vi "APX Monitor EPICS.vi"() -> ()   [LabVIEW 2015]
uses:
  <vilib>/Platform/TimedLoop/XDataNode/timing_clust.ctl
  <vilib>/Platform/TimedLoop/XDataNode/nitl_modes.ctl
  <vilib>/Platform/TimedLoop/XDataNode/wakeup.ctl
  <userlib>/caLab/Private/Get_PV-1D.vi
  <userlib>/caLab/Private/Put_I16-1D_PV-1D.vi
  <vilib>/platform/TimedLoop/XDataNode/XDataNode.xnode
  <vilib>/Platform/TimedLoop/XDataNode/XDNodeRunTimeDep.lvlib
panel:
  out "L2Turbo_ST":bool
  out "AP2Turbo_ST":bool
  out "HEMTurbo_ST":bool
  out "String":string
  out "APX:PREP_ILK":bool
  in  "OFFLINE/ONLINE":bool
  in  "APX_V1_CLOSE":bool
  in  "APX_V1_OPEN":bool
  in  "APX_V2_CLOSE":bool
  in  "APX_V2_OPEN":bool
  in  "APX_V3_CLOSE":bool
  in  "APX_V3_OPEN":bool
  in  "APX_V5_CLOSE":bool
  in  "APX_V5_OPEN":bool
  in  "APX_V4_CLOSE":bool
  in  "APX_V4_OPEN":bool
  in  "APX:Omniax:.VELO":dbl
  in  "APX:Omniax.ACCL":dbl
  in  "APX:OmniaxZ.SPMG":bool
  in  "APX:OmniaxZ.VAL":dbl
  in  "APX:Omniax:.TWV":dbl
  in  "APX:OmniaxX.TWR":bool
  in  "APX:OmniaxX.TWF":bool
  in  "APX:OmniaxY:.VELO":dbl
  in  "APX:OmniaxY.ACCL":dbl
  in  "APX:OmniaxY.SPMG":bool
  in  "APX:OmniaxY.VAL":dbl
  in  "APX:Omniaxy:.TWV":dbl
  in  "APX:OmniaxY.TWR":bool
  in  "APX:OmniaxY.TWF":bool
  in  "APX:OmniaxX:.VELO":dbl
  in  "APX:OmniaxX.ACCL":dbl
  in  "APX:OmniaxX.SPMG":bool
  in  "APX:OmniaxX.VAL":dbl
  in  "APX:Omniaxx:.TWV":dbl
  in  "APX:OmniaxX.TWR":bool
  in  "APX:OmniaxX.TWF":bool
  out "BL13-2:IG1Pressure":dbl format="%.2e"
  out "APX:HEMTurboF":dbl
  out "APX:HEMTurboP":dbl
  out "APX:HEMturboS":string
  out "APX:L2TurboF":dbl
  out "APX:L2TurboP":dbl
  out "APX:L2TurboS":string
  out "APX:AP2TurboF":dbl
  out "APX:AP2TurboP":dbl
  out "APX:AP2TurboS":string
  out "APX:V3_ENB":bool
  out "APX:V3_OPEN_REQ":bool
  out "APX:V3_SCL":bool
  out "APX:V3_SOP":bool
  out "BL132_ILK":bool
  out "SES-100_ILK":bool
  in  "loop":u8
  out "APX:V2_ENB":bool
  out "APX:V5_ENB":bool
  out "APX:V1_ENB":bool
  out "APX:V7_ENB":bool
  out "APX:V0_ENB":bool
  out "APX:V6_ENB":bool
  out "APX:V4_ENB":bool
  out "APX:V5_OPEN_REQ":bool
  out "APX:V2_OPEN_REQ":bool
  out "APX:V1_OPEN_REQ":bool
  in  "APX:V6_OPEN_REQ":bool
  out "APX:V4_OPEN_REQ":bool
  in  "APX:V0_OPEN_REQ":bool
  in  "APX:V7_OPEN_REQ":bool
  out "APX:V7_SCL":bool
  out "APX:V7_SOP":bool
  out "APX:V0_SCL":bool
  out "APX:V0_SOP":bool
  out "APX:V5_SCL":bool
  out "APX:V5_SOP":bool
  out "APX:V1_SCL":bool
  out "APX:V1_SOP":bool
  out "APX:V6_SCL":bool
  out "APX:V6_SOP":bool
  out "APX:V4_SCL":bool
  out "APX:V4_SOP":bool
  out "APX:V2_SCL":bool
  out "APX:V2_SOP":bool
  out "APX:PiezoZ":dbl format="%#_3g"
  out "APX:PiezoY":dbl format="%#_3g"
  out "APX:PiezoX":dbl format="%#_3g"
  out "APX:OmniaxX":dbl format="%#_5g"
  out "APX:OmniaxY":dbl format="%#_5g"
  out "APX:OmniaxZ.RBV":dbl
  out "BL132:132WRG1":dbl format="%.2e"
  out "APX:HPC":dbl format="%.2e"
  out "APX:Tsample":dbl format="%.1f"
  out "APX:Tpiezo":dbl format="%.1f"
  out "APX:Thpc":dbl format="%.1f"
  out "APX LEN2":dbl format="%.2e"
  out "APX:AP2":dbl format="%.2e"
  out "APX:AP1":dbl format="%.2e"
  out "APX:PREP":dbl format="%.2e"
  out "APX:HPC100":dbl format="%.4f"
  in  "stop":bool
  out "APX:HPC01":dbl format="%.6g"
  # "APX EPICS"
  # "HEMTurbo"
  # "4"
  # "SES-100 Analyzer"
  # "300l/s"
  # "L2Turbo"
  # "70l/s"
  # "3"
  # "300l/s"
  # "AP2Turbo"
  # "2"
  # "500l/s"
  # "5"
  # "300l/s"
  # "BPTrubo"
  # "AP1Turbo"
  # "1"
  # "70l/s"
  # "300l/s"
  # "70l/s"
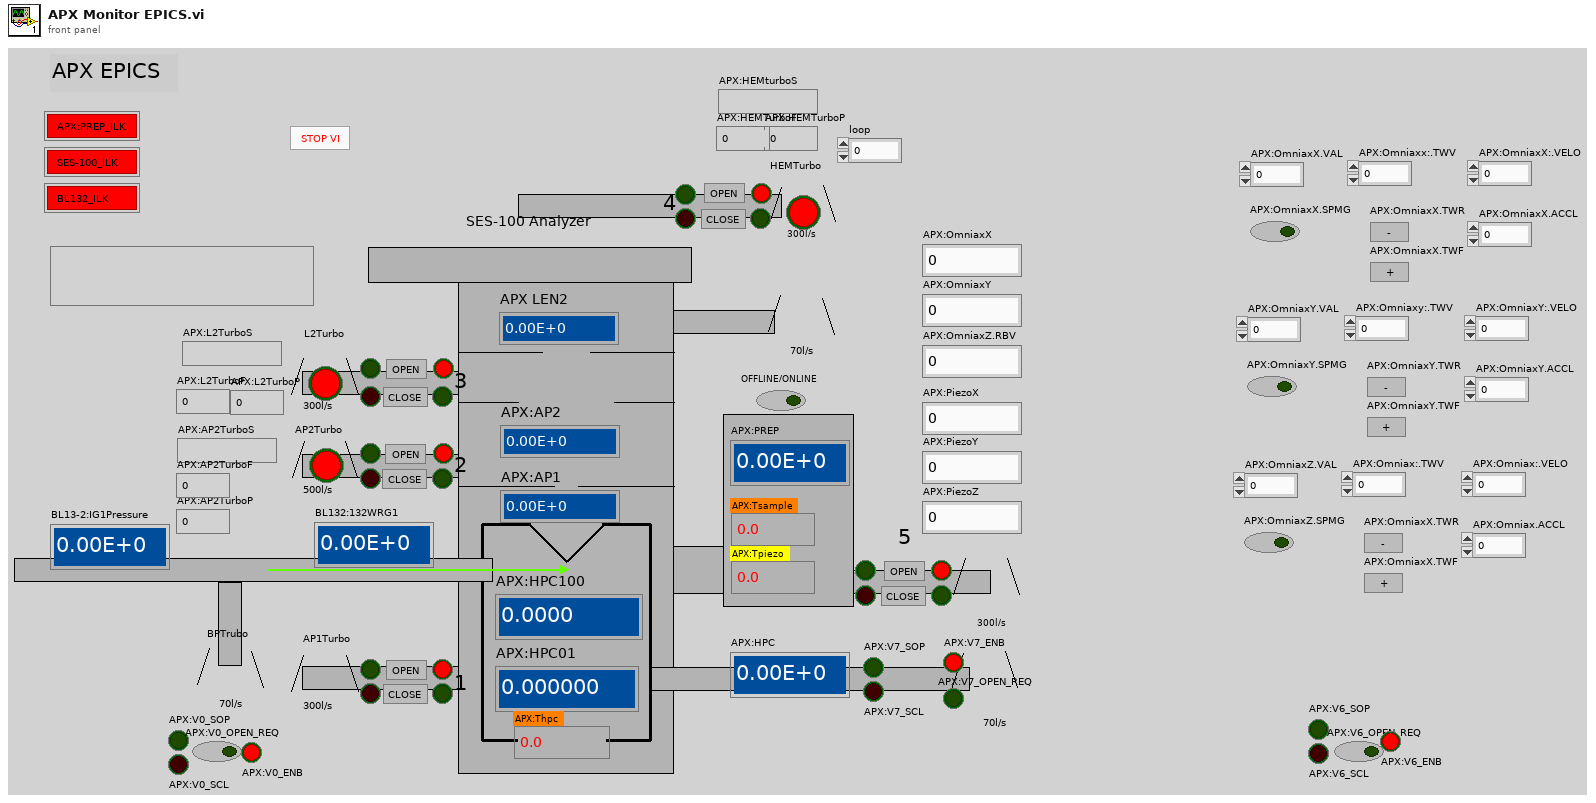
[diagram p1: front panel]
types:
  T1 = typedef "XDNodeRunTimeDep.lvlib/timing_clust.ctl" = cluster{"Expected End [f-1]":u64, "Actual End [f-1]":u64, "Finished Late? [f-1]":bool, "Expected End [i-1]":u64, "Actual End [i-1]":u64, "Finished Late? [i-1]":bool, "Expected Start [i]":u64, "Actual Start [i]":u64, "Expected Start [f]":u64, "Actual Start [f]":u64, "Source Name":string, "Structure Name":string, "Period":i64, "Deadline":i64, "Offset":i64, "Start":i64, "Priority":i32, "Timeout":i32, "Mode":T2, "Wakeup Reason":T3, "Error":errorcluster, "Source Type":string, "Secondary Source Type":string, "Global End Time":u64, "Global Start Time":u64, "Frame Duration":u64, "Iteration Duration":u64, "Assigned CPU":i32, "I/O Scan Engine Mode":u32}
  T2 = typedef "XDNodeRunTimeDep.lvlib/nitl_modes.ctl" = enum32{"No Change", "Process missed periods, maintain original phase", "Discard missed periods, maintain original phase", "Process missed periods, ignore original phase", "Discard missed periods, ignore original phase"}
  T3 = typedef "XDNodeRunTimeDep.lvlib/wakeup.ctl" = enum32{"Normal", "Aborted", "Asynchronous wakeup", "Timing source error", "Timed loop error", "Timeout"}
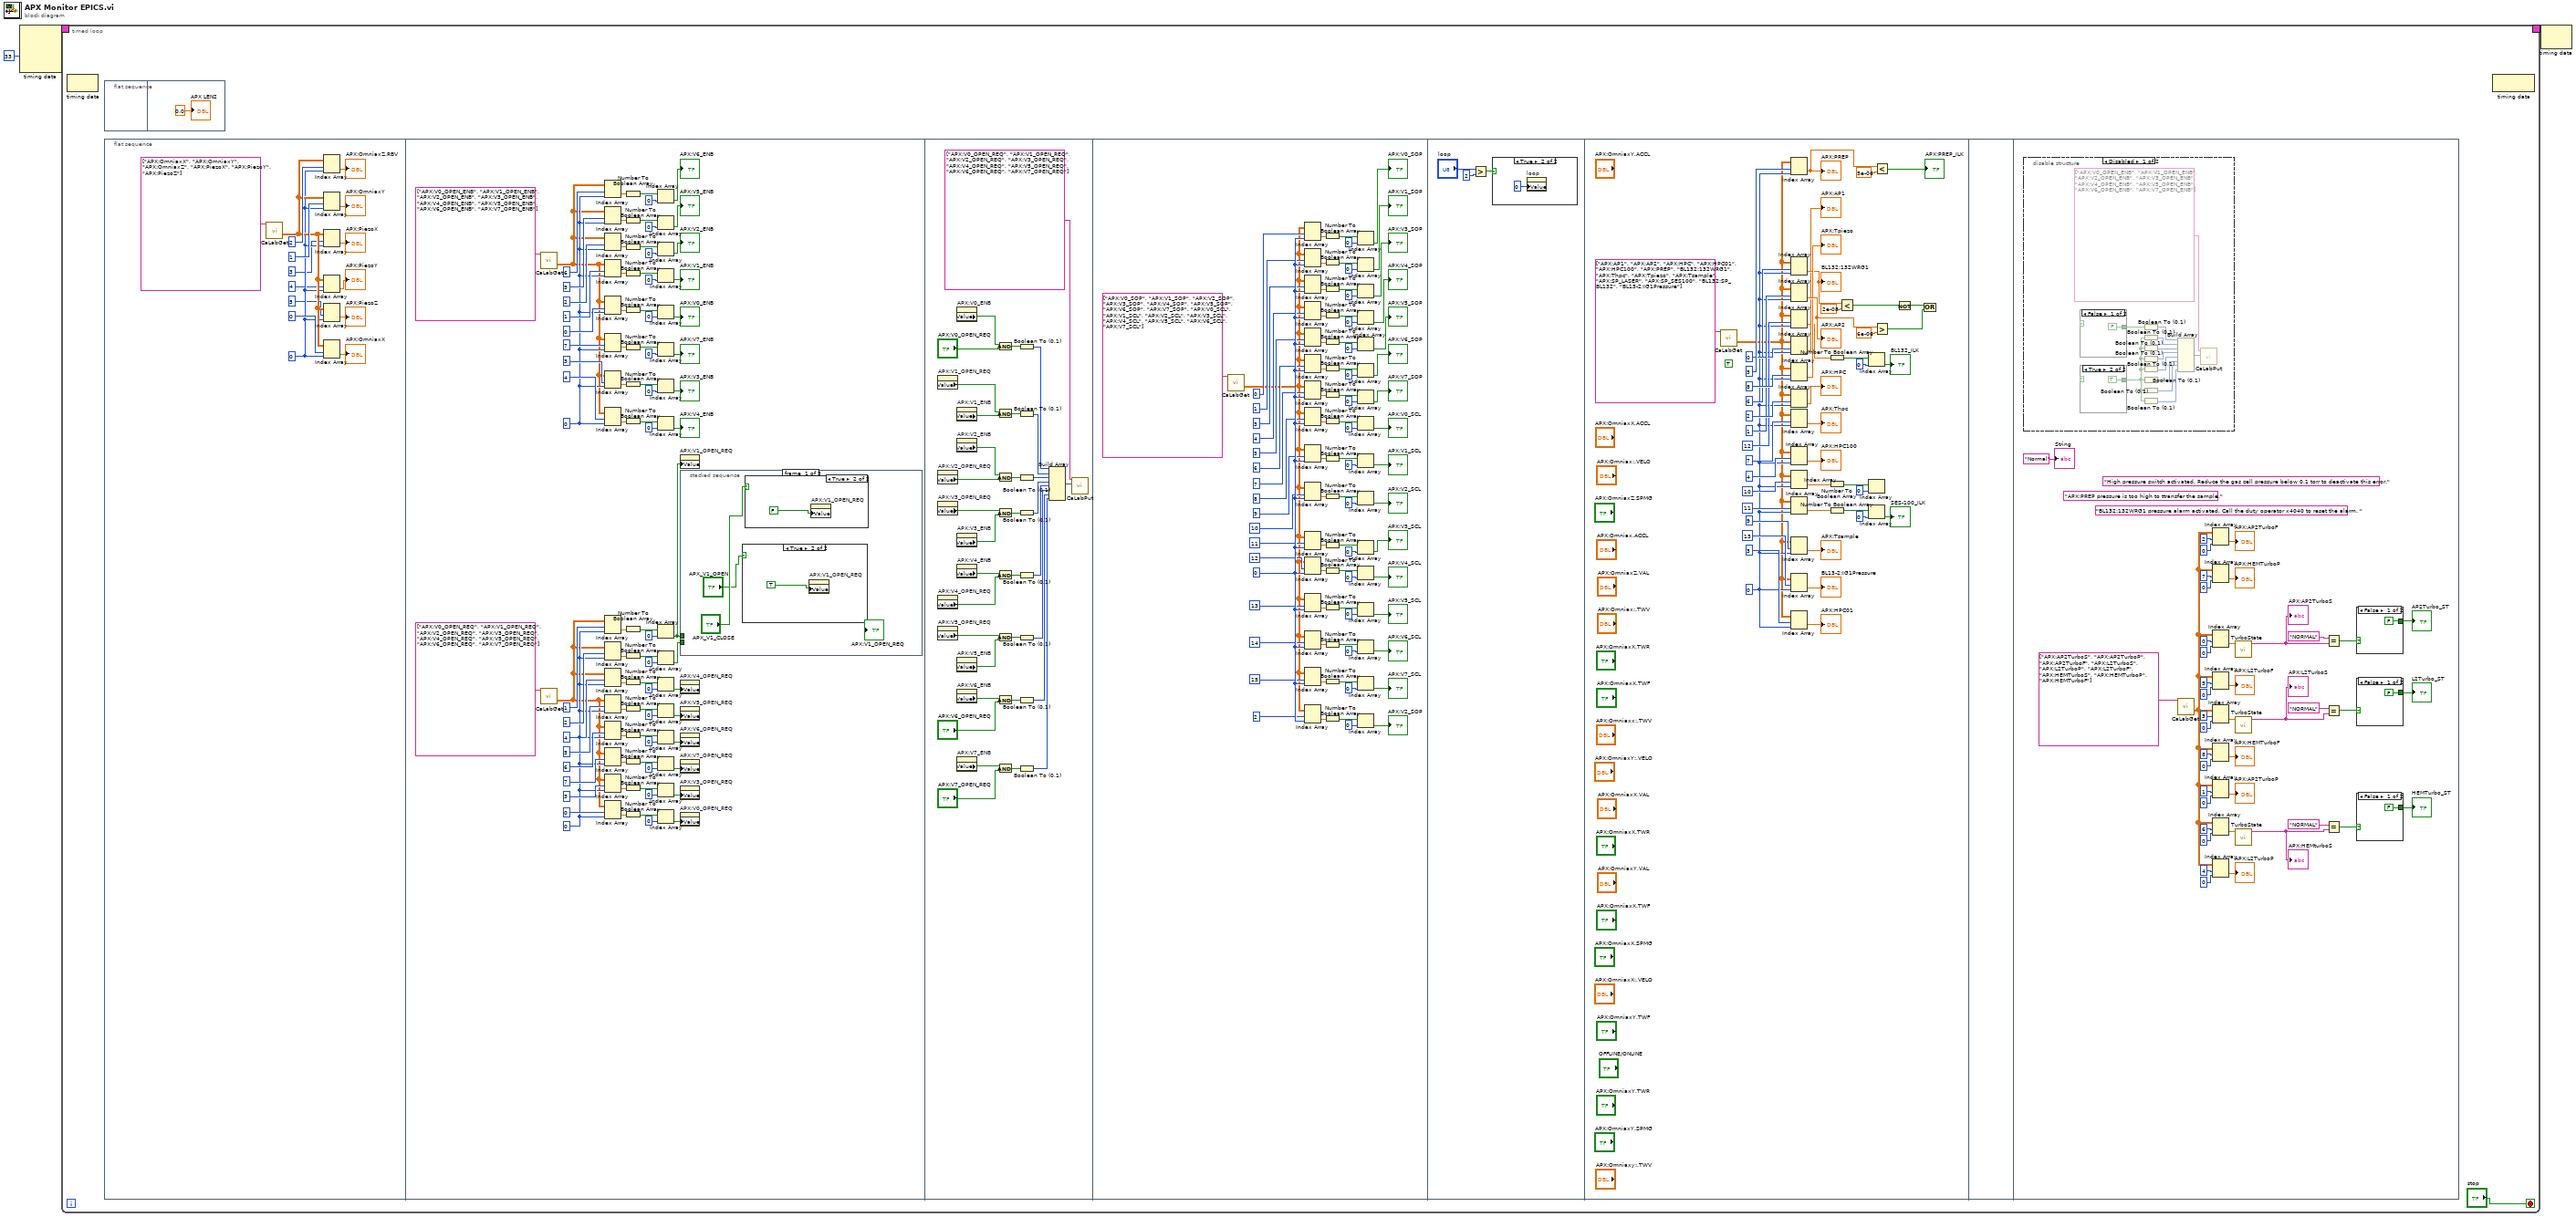
[diagram p0: block diagram]
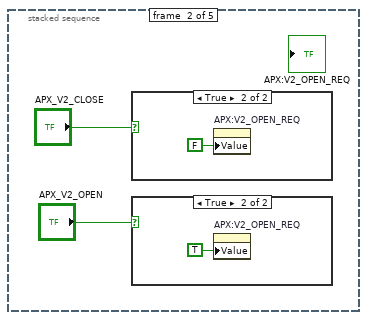
[diagram p4: hidden frame]
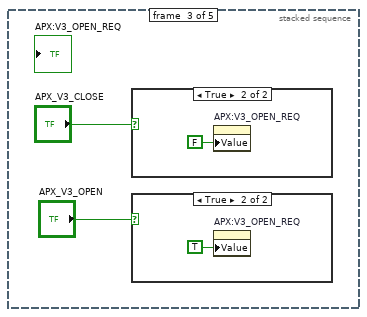
[diagram p7: hidden frame]
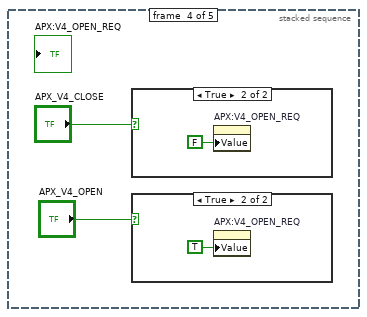
[diagram p10: hidden frame]
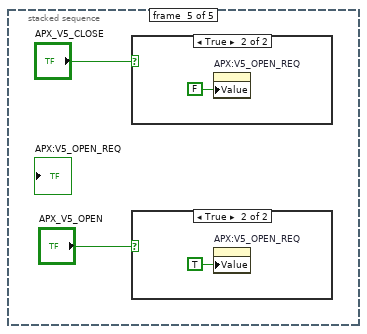
[diagram p13: hidden frame]
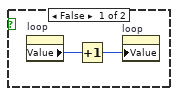
[diagram p16: hidden frame]
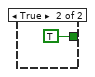
[diagram p17: hidden frame]
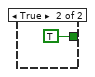
[diagram p18: hidden frame]
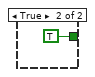
[diagram p19: hidden frame]
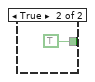
[diagram p20: hidden frame]
diagram:
  n1 = node-c288(33 ("Priority")) -> (w3:T1)  [unwired: 3 in]
  n2 = timed-loop {
    timing: w3 -> [_]
    timing-out: [_] -> w2
    stop <- "stop" stop-if-true
    n3 = node-c288() -> ()  [unwired: 1 in, 1 out]
    n4 = flat-sequence {
      frame #0 {
      }
      frame #1 {
        "APX LEN2" <- 0.0 ("APX LEN2")
      }
    }
    n5 = flat-sequence {
      frame #0 {
        w11 = 0 ("index")
        n6 = call-poly "CaLabGet.vi"("PV Names"=string[] ["APX:OmniaxX", "APX:OmniaxY", "APX:OmniaxZ", "APX:PiezoX", "APX:PiezoY", "APX:PiezoZ"]) -> ("Value Array (number)"=w12:dbl[][])  [unwired: 8 in, 6 out]
        n7 = Index Array(array=w12, index (row)=2, index (col)=w11) -> (element=→"APX:OmniaxZ.RBV":dbl)
        n8 = Index Array(array=w12, index (row)=1, index (col)=w11) -> (element=→"APX:OmniaxY":dbl)
        n9 = Index Array(array=w12, index (row)=3 ("disabled index (row)"), index (col)=w11) -> (element=→"APX:PiezoX":dbl)
        n10 = Index Array(array=w12, index (row)=4 ("disabled index (row)"), index (col)=w11) -> (element=→"APX:PiezoY":dbl)
        n11 = Index Array(array=w12, index (row)=5 ("disabled index (row)"), index (col)=w11) -> (element=→"APX:PiezoZ":dbl)
        n12 = Index Array(array=w12, index (row)=0, index (col)=w11) -> (element=→"APX:OmniaxX":dbl)
      }
      frame #1 {
        w53 = 0 ("index")
        w97 = 0 ("index")
        n13 = call-poly "CaLabGet.vi"("PV Names"=string[] ["APX:V0_OPEN_ENB", "APX:V1_OPEN_ENB", "APX:V2_OPEN_ENB", "APX:V3_OPEN_ENB", "APX:V4_OPEN_ENB", "APX:V5_OPEN_ENB", "APX:V6_OPEN_ENB", "APX:V7_OPEN_ENB"]) -> ("Value Array (number)"=w96:dbl[][])  [unwired: 8 in, 6 out]
        n14 = call-poly "CaLabGet.vi"("PV Names"=string[] ["APX:V0_OPEN_REQ", "APX:V1_OPEN_REQ", "APX:V2_OPEN_REQ", "APX:V3_OPEN_REQ", "APX:V4_OPEN_REQ", "APX:V5_OPEN_REQ", "APX:V6_OPEN_REQ", "APX:V7_OPEN_REQ"]) -> ("Value Array (number)"=w52:dbl[][])  [unwired: 8 in, 6 out]
        n15 = Index Array(array=w96, index (row)=6, index (col)=w97) -> (element=w73:dbl)
        n16 = Index Array(array=w96, index (row)=5, index (col)=w97) -> (element=w74:dbl)
        n17 = Index Array(array=w96, index (row)=2, index (col)=w97) -> (element=w77:dbl)
        n18 = Index Array(array=w96, index (row)=1, index (col)=w97) -> (element=w78:dbl)
        n19 = Index Array(array=w96, index (row)=0 ("disabled index (row)"), index (col)=w97) -> (element=w79:dbl)
        n20 = Index Array(array=w96, index (row)=7, index (col)=w97) -> (element=w72:dbl)
        n21 = Index Array(array=w96, index (row)=3, index (col)=w97) -> (element=w76:dbl)
        n22 = Index Array(array=w96, index (row)=4, index (col)=w97) -> (element=w75:dbl)
        n23 = Index Array(array=w52, index (row)=1, index (col)=w53) -> (element=w34:dbl)
        n24 = Index Array(array=w52, index (row)=2, index (col)=w53) -> (element=w33:dbl)
        n25 = Index Array(array=w52, index (row)=4, index (col)=w53) -> (element=w31:dbl)
        n26 = Index Array(array=w52, index (row)=5, index (col)=w53) -> (element=w30:dbl)
        n27 = Index Array(array=w52, index (row)=6, index (col)=w53) -> (element=w29:dbl)
        n28 = Index Array(array=w52, index (row)=7, index (col)=w53) -> (element=w28:dbl)
        n29 = Index Array(array=w52, index (row)=3, index (col)=w53) -> (element=w32:dbl)
        n30 = Index Array(array=w52, index (row)=0 ("disabled index (row)"), index (col)=w53) -> (element=w35:dbl)
        n31 = Number To Boolean Array(number=w73) -> (Boolean array=w83:bool[])
        n32 = Number To Boolean Array(number=w74) -> (Boolean array=w85:bool[])
        n33 = Number To Boolean Array(number=w77) -> (Boolean array=w91:bool[])
        n34 = Number To Boolean Array(number=w78) -> (Boolean array=w93:bool[])
        n35 = Number To Boolean Array(number=w79) -> (Boolean array=w95:bool[])
        n36 = Number To Boolean Array(number=w72) -> (Boolean array=w81:bool[])
        n37 = Number To Boolean Array(number=w76) -> (Boolean array=w89:bool[])
        n38 = Number To Boolean Array(number=w75) -> (Boolean array=w87:bool[])
        n39 = Number To Boolean Array(number=w34) -> (Boolean array=w49:bool[])
        n40 = Number To Boolean Array(number=w33) -> (Boolean array=w47:bool[])
        n41 = Number To Boolean Array(number=w31) -> (Boolean array=w43:bool[])
        n42 = Number To Boolean Array(number=w30) -> (Boolean array=w41:bool[])
        n43 = Number To Boolean Array(number=w29) -> (Boolean array=w39:bool[])
        n44 = Number To Boolean Array(number=w28) -> (Boolean array=w37:bool[])
        n45 = Number To Boolean Array(number=w32) -> (Boolean array=w45:bool[])
        n46 = Number To Boolean Array(number=w35) -> (Boolean array=w51:bool[])
        n47 = Index Array(array=w83, index=0) -> (element=→"APX:V6_ENB":bool)
        n48 = Index Array(array=w85, index=0) -> (element=→"APX:V5_ENB":bool)
        n49 = Index Array(array=w91, index=0) -> (element=→"APX:V2_ENB":bool)
        n50 = Index Array(array=w93, index=0) -> (element=→"APX:V1_ENB":bool)
        n51 = Index Array(array=w95, index=0) -> (element=→"APX:V0_ENB":bool)
        n52 = Index Array(array=w81, index=0) -> (element=→"APX:V7_ENB":bool)
        n53 = Index Array(array=w89, index=0) -> (element=→"APX:V3_ENB":bool)
        n54 = Index Array(array=w87, index=0) -> (element=→"APX:V4_ENB":bool)
        n55 = Index Array(array=w49, index=0) -> (element=w20:bool)
        n56 = Index Array(array=w47, index=0) -> (element=w21:bool)
        n57 = Index Array(array=w43, index=0) -> (element=w26:bool)
        n58 = Index Array(array=w41, index=0) -> (element=w25:bool)
        n59 = Index Array(array=w39, index=0) -> (element=w24:bool)
        n60 = Index Array(array=w37, index=0) -> (element=w23:bool)
        n61 = Index Array(array=w45, index=0) -> (element=w22:bool)
        n62 = Index Array(array=w51, index=0) -> (element=w27:bool)
        n63 = property on="APX:V1_OPEN_REQ" class="Bool (strict)"("Value"=w20) -> ()  [unwired: 2 in, 2 out]
        n64 = stacked-sequence {
          tunnel: w21 -> [_ _ _ _ _]
          tunnel: w20 -> [_ _ _ _ _]
          frame #0 {
            n65 = case shown="True" "APX_V1_OPEN" {
              frame False {
              }
              frame True {
                n66 = property on="APX:V1_OPEN_REQ" class="Bool (strict)"("Value"=TRUE ("APX:V4_OPEN_REQ")) -> ()  [unwired: 2 in, 2 out]
              }
            }
            n67 = case shown="True" "APX_V1_CLOSE" {
              frame False {
              }
              frame True {
                n68 = property on="APX:V1_OPEN_REQ" class="Bool (strict)"("Value"=FALSE ("APX:V4_OPEN_REQ")) -> ()  [unwired: 2 in, 2 out]
              }
            }
          }
          frame #1 {
            n69 = case shown="True" "APX_V2_CLOSE" {
              frame False {
              }
              frame True {
                n70 = property on="APX:V2_OPEN_REQ" class="Bool (strict)"("Value"=FALSE ("APX:V4_OPEN_REQ")) -> ()  [unwired: 2 in, 2 out]
              }
            }
            n71 = case shown="True" "APX_V2_OPEN" {
              frame False {
              }
              frame True {
                n72 = property on="APX:V2_OPEN_REQ" class="Bool (strict)"("Value"=TRUE ("APX:V4_OPEN_REQ")) -> ()  [unwired: 2 in, 2 out]
              }
            }
          }
          frame #2 {
            n73 = case shown="True" "APX_V3_CLOSE" {
              frame False {
              }
              frame True {
                n74 = property on="APX:V3_OPEN_REQ" class="Bool (strict)"("Value"=FALSE ("APX:V4_OPEN_REQ")) -> ()  [unwired: 2 in, 2 out]
              }
            }
            n75 = case shown="True" "APX_V3_OPEN" {
              frame False {
              }
              frame True {
                n76 = property on="APX:V3_OPEN_REQ" class="Bool (strict)"("Value"=TRUE ("APX:V4_OPEN_REQ")) -> ()  [unwired: 2 in, 2 out]
              }
            }
          }
          frame #3 {
            n77 = case shown="True" "APX_V4_CLOSE" {
              frame False {
              }
              frame True {
                n78 = property on="APX:V4_OPEN_REQ" class="Bool (strict)"("Value"=FALSE ("APX:V4_OPEN_REQ")) -> ()  [unwired: 2 in, 2 out]
              }
            }
            n79 = case shown="True" "APX_V4_OPEN" {
              frame False {
              }
              frame True {
                n80 = property on="APX:V4_OPEN_REQ" class="Bool (strict)"("Value"=TRUE ("APX:V4_OPEN_REQ")) -> ()  [unwired: 2 in, 2 out]
              }
            }
          }
          frame #4 {
            n81 = case shown="True" "APX_V5_CLOSE" {
              frame False {
              }
              frame True {
                n82 = property on="APX:V5_OPEN_REQ" class="Bool (strict)"("Value"=FALSE ("APX:V4_OPEN_REQ")) -> ()  [unwired: 2 in, 2 out]
              }
            }
            n83 = case shown="True" "APX_V5_OPEN" {
              frame False {
              }
              frame True {
                n84 = property on="APX:V5_OPEN_REQ" class="Bool (strict)"("Value"=TRUE ("APX:V4_OPEN_REQ")) -> ()  [unwired: 2 in, 2 out]
              }
            }
          }
        }
        n85 = property on="APX:V4_OPEN_REQ" class="Bool (strict)"("Value"=w26) -> ()  [unwired: 2 in, 2 out]
        n86 = property on="APX:V5_OPEN_REQ" class="Bool (strict)"("Value"=w25) -> ()  [unwired: 2 in, 2 out]
        n87 = property on="APX:V6_OPEN_REQ" class="Bool (strict)"("Value"=w24) -> ()  [unwired: 2 in, 2 out]
        n88 = property on="APX:V7_OPEN_REQ" class="Bool (strict)"("Value"=w23) -> ()  [unwired: 2 in, 2 out]
        n89 = property on="APX:V3_OPEN_REQ" class="Bool (strict)"("Value"=w22) -> ()  [unwired: 2 in, 2 out]
        n90 = property on="APX:V0_OPEN_REQ" class="Bool (strict)"("Value"=w27) -> ()  [unwired: 2 in, 2 out]
      }
      frame #2 {
        n91 = property on="APX:V1_OPEN_REQ" class="Bool (strict)"() -> ("Value"=w126:bool)  [unwired: 2 in, 2 out]
        n92 = property on="APX:V2_OPEN_REQ" class="Bool (strict)"() -> ("Value"=w127:bool)  [unwired: 2 in, 2 out]
        n93 = property on="APX:V3_OPEN_REQ" class="Bool (strict)"() -> ("Value"=w128:bool)  [unwired: 2 in, 2 out]
        n94 = property on="APX:V4_OPEN_REQ" class="Bool (strict)"() -> ("Value"=w130:bool)  [unwired: 2 in, 2 out]
        n95 = property on="APX:V5_OPEN_REQ" class="Bool (strict)"() -> ("Value"=w129:bool)  [unwired: 2 in, 2 out]
        n96 = property on="APX:V0_ENB" class="Bool (strict)"() -> ("Value"=w138:bool)  [unwired: 2 in, 2 out]
        n97 = property on="APX:V1_ENB" class="Bool (strict)"() -> ("Value"=w137:bool)  [unwired: 2 in, 2 out]
        n98 = property on="APX:V2_ENB" class="Bool (strict)"() -> ("Value"=w136:bool)  [unwired: 2 in, 2 out]
        n99 = property on="APX:V3_ENB" class="Bool (strict)"() -> ("Value"=w131:bool)  [unwired: 2 in, 2 out]
        n100 = property on="APX:V4_ENB" class="Bool (strict)"() -> ("Value"=w135:bool)  [unwired: 2 in, 2 out]
        n101 = property on="APX:V5_ENB" class="Bool (strict)"() -> ("Value"=w134:bool)  [unwired: 2 in, 2 out]
        n102 = property on="APX:V6_ENB" class="Bool (strict)"() -> ("Value"=w133:bool)  [unwired: 2 in, 2 out]
        n103 = property on="APX:V7_ENB" class="Bool (strict)"() -> ("Value"=w132:bool)  [unwired: 2 in, 2 out]
        n104 = And(x=w138, y="APX:V0_OPEN_REQ") -> (x .and. y?=w146:bool)
        n105 = And(x=w126, y=w137) -> (x .and. y?=w145:bool)
        n106 = And(x=w136, y=w127) -> (x .and. y?=w144:bool)
        n107 = And(x=w128, y=w131) -> (x .and. y?=w143:bool)
        n108 = And(x=w135, y=w130) -> (x .and. y?=w142:bool)
        n109 = And(x=w129, y=w134) -> (x .and. y?=w141:bool)
        n110 = And(x=w133, y="APX:V6_OPEN_REQ") -> (x .and. y?=w140:bool)
        n111 = And(x=w132, y="APX:V7_OPEN_REQ") -> (x .and. y?=w139:bool)
        n112 = Boolean To (0,1)(Boolean=w146) -> (0, 1=w156:i16)
        n113 = Boolean To (0,1)(Boolean=w145) -> (0, 1=w155:i16)
        n114 = Boolean To (0,1)(Boolean=w144) -> (0, 1=w154:i16)
        n115 = Boolean To (0,1)(Boolean=w143) -> (0, 1=w153:i16)
        n116 = Boolean To (0,1)(Boolean=w142) -> (0, 1=w152:i16)
        n117 = Boolean To (0,1)(Boolean=w141) -> (0, 1=w151:i16)
        n118 = Boolean To (0,1)(Boolean=w140) -> (0, 1=w150:i16)
        n119 = Boolean To (0,1)(Boolean=w139) -> (0, 1=w149:i16)
        n120 = Build Array(w156, w155, w154, w153, w152, w151, w150, w149) -> (w148:i16[])
        n121 = call-poly <userlib>:"CaLabPut.vi"("Values"=w148, "PV Names"=string[] ["APX:V0_OPEN_REQ", "APX:V1_OPEN_REQ", "APX:V2_OPEN_REQ", "APX:V3_OPEN_REQ", "APX:V4_OPEN_REQ", "APX:V5_OPEN_REQ", "APX:V6_OPEN_REQ", "APX:V7_OPEN_REQ"]) -> ()  [unwired: 6 in, 4 out]
      }
      frame #3 {
        w180 = 0 ("index")
        n122 = call-poly "CaLabGet.vi"("PV Names"=string[] ["APX:V0_SOP", "APX:V1_SOP", "APX:V2_SOP", "APX:V3_SOP", "APX:V4_SOP", "APX:V5_SOP", "APX:V6_SOP", "APX:V7_SOP", "APX:V0_SCL", "APX:V1_SCL", "APX:V2_SCL", "APX:V3_SCL", "APX:V4_SCL", "APX:V5_SCL", "APX:V6_SCL", "APX:V7_SCL"]) -> ("Value Array (number)"=w162:dbl[][])  [unwired: 8 in, 6 out]
        n123 = Index Array(array=w162, index (row)=0 ("disabled index (row)"), index (col)=w180) -> (element=w228:dbl)
        n124 = Index Array(array=w162, index (row)=1, index (col)=w180) -> (element=w229:dbl)
        n125 = Index Array(array=w162, index (row)=3, index (col)=w180) -> (element=w231:dbl)
        n126 = Index Array(array=w162, index (row)=4, index (col)=w180) -> (element=w232:dbl)
        n127 = Index Array(array=w162, index (row)=5, index (col)=w180) -> (element=w233:dbl)
        n128 = Index Array(array=w162, index (row)=6, index (col)=w180) -> (element=w234:dbl)
        n129 = Index Array(array=w162, index (row)=7, index (col)=w180) -> (element=w235:dbl)
        n130 = Index Array(array=w162, index (row)=8 ("disabled index (row)"), index (col)=w180) -> (element=w181:dbl)
        n131 = Index Array(array=w162, index (row)=9, index (col)=w180) -> (element=w197:dbl)
        n132 = Index Array(array=w162, index (row)=10, index (col)=w180) -> (element=w198:dbl)
        n133 = Index Array(array=w162, index (row)=11, index (col)=w180) -> (element=w199:dbl)
        n134 = Index Array(array=w162, index (row)=12, index (col)=w180) -> (element=w200:dbl)
        n135 = Index Array(array=w162, index (row)=13, index (col)=w180) -> (element=w201:dbl)
        n136 = Index Array(array=w162, index (row)=14, index (col)=w180) -> (element=w202:dbl)
        n137 = Index Array(array=w162, index (row)=15, index (col)=w180) -> (element=w205:dbl)
        n138 = Index Array(array=w162, index (row)=2, index (col)=w180) -> (element=w230:dbl)
        n139 = Number To Boolean Array(number=w228) -> (Boolean array=w212:bool[])
        n140 = Number To Boolean Array(number=w229) -> (Boolean array=w214:bool[])
        n141 = Number To Boolean Array(number=w231) -> (Boolean array=w218:bool[])
        n142 = Number To Boolean Array(number=w232) -> (Boolean array=w220:bool[])
        n143 = Number To Boolean Array(number=w233) -> (Boolean array=w222:bool[])
        n144 = Number To Boolean Array(number=w234) -> (Boolean array=w224:bool[])
        n145 = Number To Boolean Array(number=w235) -> (Boolean array=w226:bool[])
        n146 = Number To Boolean Array(number=w181) -> (Boolean array=w182:bool[])
        n147 = Number To Boolean Array(number=w197) -> (Boolean array=w185:bool[])
        n148 = Number To Boolean Array(number=w198) -> (Boolean array=w187:bool[])
        n149 = Number To Boolean Array(number=w199) -> (Boolean array=w189:bool[])
        n150 = Number To Boolean Array(number=w200) -> (Boolean array=w191:bool[])
        n151 = Number To Boolean Array(number=w201) -> (Boolean array=w193:bool[])
        n152 = Number To Boolean Array(number=w202) -> (Boolean array=w195:bool[])
        n153 = Number To Boolean Array(number=w205) -> (Boolean array=w203:bool[])
        n154 = Number To Boolean Array(number=w230) -> (Boolean array=w216:bool[])
        n155 = Index Array(array=w212, index=0) -> (element=→"APX:V0_SOP":bool)
        n156 = Index Array(array=w214, index=0) -> (element=→"APX:V1_SOP":bool)
        n157 = Index Array(array=w218, index=0) -> (element=→"APX:V3_SOP":bool)
        n158 = Index Array(array=w220, index=0) -> (element=→"APX:V4_SOP":bool)
        n159 = Index Array(array=w222, index=0) -> (element=→"APX:V5_SOP":bool)
        n160 = Index Array(array=w224, index=0) -> (element=→"APX:V6_SOP":bool)
        n161 = Index Array(array=w226, index=0) -> (element=→"APX:V7_SOP":bool)
        n162 = Index Array(array=w182, index=0) -> (element=→"APX:V0_SCL":bool)
        n163 = Index Array(array=w185, index=0) -> (element=→"APX:V1_SCL":bool)
        n164 = Index Array(array=w187, index=0) -> (element=→"APX:V2_SCL":bool)
        n165 = Index Array(array=w189, index=0) -> (element=→"APX:V3_SCL":bool)
        n166 = Index Array(array=w191, index=0) -> (element=→"APX:V4_SCL":bool)
        n167 = Index Array(array=w193, index=0) -> (element=→"APX:V5_SCL":bool)
        n168 = Index Array(array=w195, index=0) -> (element=→"APX:V6_SCL":bool)
        n169 = Index Array(array=w203, index=0) -> (element=→"APX:V7_SCL":bool)
        n170 = Index Array(array=w216, index=0) -> (element=→"APX:V2_SOP":bool)
      }
      frame #4 {
        n171 = Greater?(x="loop", y=u8 2) -> (0:w245:bool)
        n172 = case shown="True" w245 {
          frame False {
            n173 = property on="loop" class="DigNum (strict)"() -> ("Value"=w246:u8)  [unwired: 2 in, 2 out]
            n174 = Increment(x=w246) -> (x+1=w247:u8)
            n175 = property on="loop" class="DigNum (strict)"("Value"=w247) -> ()  [unwired: 2 in, 2 out]
          }
          frame True {
            n176 = property on="loop" class="DigNum (strict)"("Value"=u8 0 ("loop")) -> ()  [unwired: 2 in, 2 out]
          }
        }
      }
      frame #5 {
        w254 = 0 ("index")
        (unwired) TRUE ("x")
        n177 = call-poly "CaLabGet.vi"("PV Names"=string[] ["APX:AP1", "APX:AP2", "APX:HPC", "APX:HPC01", "APX:HPC100", "APX:PREP", "BL132:132WRG1", "APX:Thpc", "APX:Tpiezo", "APX:Tsample", "APX:SP_LASER", "APX:SP_SES100", "BL132:SP_BL132", "BL13-2:IG1Pressure"]) -> ("Value Array (number)"=w253:dbl[][])  [unwired: 8 in, 6 out]
        n178 = Index Array(array=w253, index (row)=5, index (col)=w254) -> (element=w251:dbl)
        "APX:PREP" <- w251
        n179 = Index Array(array=w253, index (row)=6 ("index"), index (col)=w254) -> (element=w283:dbl)
        "BL132:132WRG1" <- w283
        n180 = Index Array(array=w253, index (row)=1 ("disabled index (row)"), index (col)=w254) -> (element=w292:dbl)
        "APX:AP2" <- w292
        n181 = Index Array(array=w253, index (row)=12, index (col)=w254) -> (element=w258:dbl)
        n182 = Index Array(array=w253, index (row)=0, index (col)=w254) -> (element=→"APX:AP1":dbl)
        n183 = Index Array(array=w253, index (row)=8, index (col)=w254) -> (element=→"APX:Tpiezo":dbl)
        n184 = Index Array(array=w253, index (row)=2, index (col)=w254) -> (element=→"APX:HPC":dbl)
        n185 = Index Array(array=w253, index (row)=7, index (col)=w254) -> (element=→"APX:Thpc":dbl)
        n186 = Index Array(array=w253, index (row)=4, index (col)=w254) -> (element=→"APX:HPC100":dbl)
        n187 = Index Array(array=w253, index (row)=10, index (col)=w254) -> (element=w266:dbl)
        n188 = Index Array(array=w253, index (row)=11, index (col)=w254) -> (element=w261:dbl)
        n189 = Index Array(array=w253, index (row)=9, index (col)=w254) -> (element=→"APX:Tsample":dbl)
        n190 = Index Array(array=w253, index (row)=13, index (col)=w254) -> (element=→"BL13-2:IG1Pressure":dbl)
        n191 = Index Array(array=w253, index (row)=3, index (col)=w254) -> (element=→"APX:HPC01":dbl)
        n192 = Number To Boolean Array(number=w258) -> (Boolean array=w260:bool[])
        n193 = Number To Boolean Array(number=w266) -> (Boolean array=w265:bool[])
        n194 = Number To Boolean Array(number=w261) -> (Boolean array=w263:bool[])
        n195 = Less?(x=w283, y=2e-08) -> (x < y?=w290:bool)
        n196 = Index Array(array=w260, index=0) -> (element=→"BL132_ILK":bool)
        n197 = Index Array(array=w265, index=0) -> ()  [unwired: 1 out]
        n198 = Index Array(array=w263, index=0) -> (element=→"SES-100_ILK":bool)
        n199 = Less?(x=w251, y=5e-06) -> (x < y?=→"APX:PREP_ILK":bool)
        n200 = Greater?(x=w292, y=6e-06) -> (0:w294:bool)
        n201 = Not(x=w290) -> (.not. x?=w293:bool)
        n202 = Or(x=w293, y=w294) -> ()  [unwired: 1 out]
      }
      frame #6 {
      }
      frame #7 {
        (unwired) "APX:PREP pressure is too high to ttransfer the sample." ("Message")
        (unwired) "BL132:132WRG1 pressure alarm activated. Call the duty operator x4040 to reset the alarm. " ("Message")
        (unwired) "High pressure switch activated. Reduce the gas cell pressure below 0.1 torr to deactivate this error." ("Message")
        n203 = disable-structure shown="Disabled" {
          frame Disabled {
            n204 = case shown="False" {
              selector: _ -> [_ _]
              tunnel: [FALSE TRUE] -> w344
              frame False {
              }
              frame True {
              }
            }
            n205 = case shown="True" {
              selector: _ -> [_ _]
              tunnel: [FALSE TRUE] -> w343
              frame False {
              }
              frame True {
              }
            }
            n206 = Boolean To (0,1)(Boolean=w344) -> (0, 1=w354:i16)
            n207 = Boolean To (0,1)(Boolean=w343) -> (0, 1=w353:i16)
            n208 = Boolean To (0,1)(Boolean=w343) -> (0, 1=w352:i16)
            n209 = Boolean To (0,1)(Boolean=w343) -> (0, 1=w351:i16)
            n210 = Boolean To (0,1)(Boolean=w343) -> (0, 1=w350:i16)
            n211 = Boolean To (0,1)(Boolean=w343) -> (0, 1=w349:i16)
            n212 = Boolean To (0,1)(Boolean=w343) -> (0, 1=w348:i16)
            n213 = Boolean To (0,1)(Boolean=w343) -> (0, 1=w347:i16)
            n214 = Build Array(w354, w353, w352, w351, w350, w349, w348, w347) -> (w346:i16[])
            n215 = call-poly <userlib>:"CaLabPut.vi"("Values"=w346, "PV Names"=string[] ["APX:V0_OPEN_ENB", "APX:V1_OPEN_ENB", "APX:V2_OPEN_ENB", "APX:V3_OPEN_ENB", "APX:V4_OPEN_ENB", "APX:V5_OPEN_ENB", "APX:V6_OPEN_ENB", "APX:V7_OPEN_ENB"]) -> ()  [unwired: 6 in, 4 out]
          }
          frame Enabled {
          }
        }
        n216 = call-poly "CaLabGet.vi"("PV Names"=string[] ["APX:AP2TurboS", "APX:AP2TurboP", "APX:AP2TurboF", "APX:L2TurboS", "APX:L2TurboP", "APX:L2TurboF", "APX:HEMTurboS", "APX:HEMTurboP", "APX:HEMTurboF"]) -> ("Value Array (number)"=w321:dbl[][])  [unwired: 8 in, 6 out]
        n217 = Index Array(array=w321, index (row)=2 ("index"), index (col)=0 ("disabled index (col)")) -> (element=→"APX:AP2TurboF":dbl)
        n218 = Index Array(array=w321, index (row)=7 ("index"), index (col)=0 ("disabled index (col)")) -> (element=→"APX:HEMTurboP":dbl)
        n219 = Index Array(array=w321, index (row)=0 ("index"), index (col)=0 ("disabled index (col)")) -> (element=w316:dbl)
        n220 = Index Array(array=w321, index (row)=5 ("index"), index (col)=0 ("disabled index (col)")) -> (element=→"APX:L2TurboF":dbl)
        n221 = Index Array(array=w321, index (row)=3 ("index"), index (col)=0 ("disabled index (col)")) -> (element=w313:dbl)
        n222 = Index Array(array=w321, index (row)=8 ("index"), index (col)=0 ("disabled index (col)")) -> (element=→"APX:HEMTurboF":dbl)
        n223 = Index Array(array=w321, index (row)=1 ("index"), index (col)=0 ("disabled index (col)")) -> (element=→"APX:AP2TurboP":dbl)
        n224 = Index Array(array=w321, index (row)=6 ("index"), index (col)=0 ("disabled index (col)")) -> (element=w310:dbl)
        n225 = Index Array(array=w321, index (row)=4 ("index"), index (col)=0 ("disabled index (col)")) -> (element=→"APX:L2TurboP":dbl)
        n226 = call "TurboState.vi"("Numeric"=w316) -> ("String"=w295:string)  [unwired: 10 in]
        "APX:AP2TurboS" <- w295
        n227 = call "TurboState.vi"("Numeric"=w313) -> ("String"=w296:string)  [unwired: 10 in]
        "APX:L2TurboS" <- w296
        n228 = call "TurboState.vi"("Numeric"=w310) -> ("String"=w306:string)  [unwired: 10 in]
        "APX:HEMturboS" <- w306
        n229 = Equal?(x="NORMAL", y=w295) -> (x = y?=w301:bool)
        n230 = Equal?(x="NORMAL", y=w296) -> (x = y?=w298:bool)
        n231 = Equal?(x="NORMAL", y=w306) -> (x = y?=w304:bool)
        n232 = case shown="False" w301 {
          tunnel: [FALSE TRUE] -> w300
          frame False {
          }
          frame True {
          }
        }
        "AP2Turbo_ST" <- w300
        n233 = case shown="False" w298 {
          tunnel: [FALSE TRUE] -> w297
          frame False {
          }
          frame True {
          }
        }
        "L2Turbo_ST" <- w297
        n234 = case shown="False" w304 {
          tunnel: [FALSE TRUE] -> w303
          frame False {
          }
          frame True {
          }
        }
        "HEMTurbo_ST" <- w303
        "String" <- "Normal" ("Message")
      }
    }
    n235 = node-c288() -> ()  [unwired: 1 in, 1 out]
  }
  n236 = node-c288(w2) -> ()  [unwired: 1 out]
